vi "test Move Channels To Engine.vi"(8 "error in (no error)":errorcluster, 11 "TestCase in":refnum<class "Configuration Tests.lvclass">) -> (0 "error out":errorcluster, 3 "TestCase out":refnum<class "Configuration Tests.lvclass">)   [LabVIEW 2017, in "Configuration Tests.lvclass"]
uses:
  Configuration Tests.lvclass
  Mock Classes/Transfer Group/Mock Transfer Group.lvclass
  C:/github/data-sharing-framework/Data Sharing Framework Core/Engine/Classes/Transfer Group/Transfer Group.lvclass
  Mock Classes/Transfer/Mock Transfer.lvclass
  C:/github/data-sharing-framework/Data Sharing Framework Core/Engine/Classes/Transfer/Transfer.lvclass
  Engine/Classes/Transfer Group/Transfer Group.lvclass/Transfer Group.ctl
  Engine/Classes/Transfer/Transfer.lvclass/Transfer.ctl
  <vilib>/NI/Memory Manager/Classes/Pointer/Pointer.lvclass/Pointer.ctl
  Engine/Classes/Pointer/DBL Pointer.lvclass/DBL Pointer.ctl
  Engine/Classes/Transfer Group/Get Transfers.vi
  Engine/Classes/Transfer/Get Inline Buffer.vi
  Engine/Classes/Transfer/Get Intermediate Buffer.vi
  <vilib>/NI/Memory Manager/Classes/Pointer/API/Copy All Pointer Data.vi
  Engine/Classes/Pointer/Get Channel Count.vi
  <vilib>/NI/Memory Manager/Classes/Pointer/API/Read Pointer Data.vi
  <vilib>/NI/Memory Manager/Classes/Pointer/Public/Read/Read (1D DBL).vi
  <vilib>/NI/Memory Manager/Classes/Pointer/API/Accessors/Get Size.vi
  <vilib>/NI/Memory Manager/Classes/Pointer/API/Copy Pointer Data.vi
  <vilib>/NI/Memory Manager/Classes/Pointer/Public/Read (No Check)/Read (No Check 1D DBL).vi
  <vilib>/NI/Memory Manager/Classes/Pointer/Protected/Parameter Checking/Check Null Pointer.vi
  <vilib>/NI/Memory Manager/Classes/Pointer/Protected/Parameter Checking/Check Subset (Power of 2).vi
  <vilib>/NI/Memory Manager/Classes/Pointer/Public/Copy (No Check).vi
  <vilib>/NI/Memory Manager/Classes/Pointer/Protected/Parameter Checking/Check Subset.vi
  <vilib>/NI/Memory Manager/Classes/Pointer/API/Accessors/Get Address.vi
  <vilib>/NI/Memory Manager/Classes/Pointer/Protected/Errors.vi
  <vilib>/NI/Memory Manager/Classes/Pointer/Protected/Error VIs/Null Pointer.vi
  <vilib>/NI/Memory Manager/Classes/Pointer/Protected/Error VIs/Out of Bounds.vi
  <vilib>/NI/Memory Manager/Classes/Pointer/Private/Count to Size.vi
  <vilib>/NI/Memory Manager/Classes/Pointer/Protected/Error Building/Create Error.vi
  <vilib>/NI/Memory Manager/VIs/Write String into Source.vi
  <vilib>/NI/Memory Manager/Classes/Pointer/Protected/Error Building/Write Pointer Size.vi
  <vilib>/NI/Memory Manager/VIs/Write Number into Source.vi
  <vilib>/NI/Memory Manager/VIs/VIs for Poly/Write U64 into Source.vi
  <vilib>/NI/Memory Manager/Constants/Constants.vi
  <vilib>/NI/Memory Manager/Constants/Library Name.vi
  <vilib>/NI/Memory Manager/Classes/Pointer/Protected/Error Building/Get Error Info.vi
  <vilib>/NI/Memory Manager/VIs/Create Error Cluster.vi
  <vilib>/NI/Memory Manager/VIs/VIs for Poly/Create Error Cluster (256B).vi
  <vilib>/NI/Memory Manager/VIs/Set Error Status.vi
  <vilib>/NI/Memory Manager/VIs/Set Error Code.vi
  <vilib>/NI/Memory Manager/VIs/Set Error Source.vi
  Engine/Classes/Pointer/DBL Pointer.lvclass
  C:/Program Files (x86)/National Instruments/LabVIEW 2017/vi.lib/NI/Memory Manager/Classes/Pointer/Pointer.lvclass
  <vilib>/addons/_JKI Toolkits/VI Tester/TestCase.llb/TestCase.lvclass
  Engine/Classes/Transfer Group/Transfer Group.lvclass
  C:/Program Files (x86)/National Instruments/LabVIEW 2017/vi.lib/addons/_JKI Toolkits/VI Tester/TestCase.llb/TestCase.lvclass
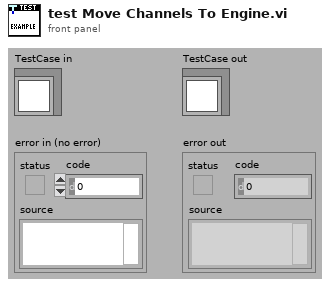
[diagram p1: front panel]
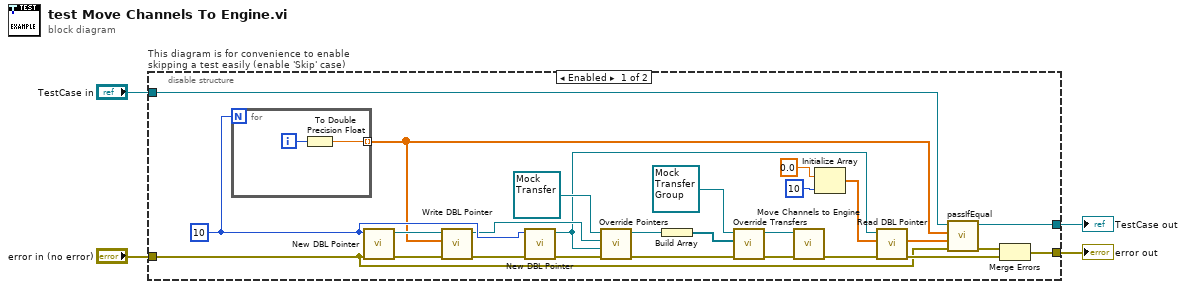
[diagram p0: block diagram]
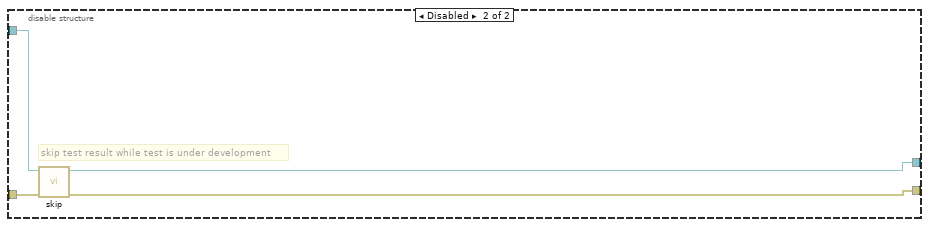
[diagram p2: hidden frame]
diagram:
  n1 = disable-structure "This diagram is for convenience to enable skipping a test easily (enable 'Skip' case)" shown="Enabled" {
    disable-tunnel: "TestCase in" -> [w16 w36]
    disable-tunnel: [w15 w34] -> w1
    disable-tunnel: [w7 w35] -> w3
    disable-tunnel: "error in (no error)" -> [w5 w33]
    frame Enabled {
      w29 = u64 10 ("channel count")
      n2 = for {
        N: w29 -> [_]
        tunnel: [w31] -> w14 mode=indexing
        i -> [w32]
        n3 = To Double Precision Float(number=w32) -> (double precision float=w31:dbl)
      }
      n4 = call "New DBL Pointer.vi"("error in (no error)"=w5, "channel count"=w29) -> ("error out"=w12:errorcluster, "DBL Pointer out"=w30:refnum<class "DBL Pointer.lvclass">)  [unwired: 8 in]
      n5 = call "Write DBL Pointer.vi"("error in (no error)"=w12, "buffer in"=w14, "DBL Pointer in"=w30) -> ("error out"=w11:errorcluster, "DBL Pointer out"=w28:refnum<class "DBL Pointer.lvclass">)  [unwired: 6 in, 1 out]
      n6 = call "New DBL Pointer.vi"("error in (no error)"=w11, "channel count"=w29) -> ("error out"=w10:errorcluster, "DBL Pointer out"=w22:refnum<class "DBL Pointer.lvclass">)  [unwired: 8 in]
      n7 = call "Override Pointers.vi"("error in (no error)"=w10, "Intermediate Buffer"=w22, "Inline Buffer"=w28, "Mock Transfer in"=refnum<class "Mock Transfer.lvclass"> refnum ("Mock Transfer.lvclass")) -> ("error out"=w9:errorcluster, "Mock Transfer out"=w26:refnum<class "Mock Transfer.lvclass">)  [unwired: 6 in]
      n8 = Build Array(w26) -> (w25:refnum<class "Mock Transfer.lvclass">[])
      n9 = call "Override Transfers.vi"("error in (no error)"=w9, "Transfers"=w25, "Mock Transfer Group in"=refnum<class "Mock Transfer Group.lvclass"> refnum ("Mock Transfer Group.lvclass")) -> ("error out"=w8:errorcluster, "Mock Transfer Group out"=w23:refnum<class "Mock Transfer Group.lvclass">)  [unwired: 7 in]
      n10 = call "Move Channels to Engine.vi"("error in (no error)"=w8, "Transfer Group in"=w23) -> ("error out"=w21:errorcluster)  [unwired: 8 in, 1 out]
      n11 = Initialize Array(0.0 ("element"), 10 ("dimension size")) -> (w19:dbl[])
      n12 = call "Read DBL Pointer.vi"("error in (no error)"=w21, "buffer in"=w19, "DBL Pointer in"=w22) -> ("error out"=w6:errorcluster, "buffer out"=w13:dbl[])  [unwired: 6 in, 1 out]
      n13 = call-dynamic "passIfEqual.vi"("error in (no error)"=w5, "y"=w13, "x"=w14, "TestCase in"=w16) -> ("error out"=w17:errorcluster, "TestCase out"=w15:refnum<class "Configuration Tests.lvclass">)  [unwired: 6 in]
      n14 = Merge Errors(w17, w6) -> (w7:errorcluster)
    }
    frame Disabled {
      # "skip test result while test is under development"
      n15 = call <vilib>:"skip.vi"("error in (no error)"=w33, "TestCase in"=w36) -> ("error out"=w35:errorcluster, "TestCase out"=w34:refnum<class "Configuration Tests.lvclass">)  [unwired: 8 in]
    }
  }
  "error out" <- w3
  "TestCase out" <- w1
